vi "Flight Timer.vi"(10 "Aircraft Speed (m/s)":dbl, 11 "System Status":string) -> (2 "Flight Time":string, 3 "Flight Time":dbl)   [LabVIEW 2014]
uses:
  Controls/Flight Timer States.ctl
  Missions/FGVs/Current Mission Distance/Methods/Get Mission Distance.vi
  Missions/FGVs/Virtual Waypoints/Methods/Get Virtual Waypoints.vi
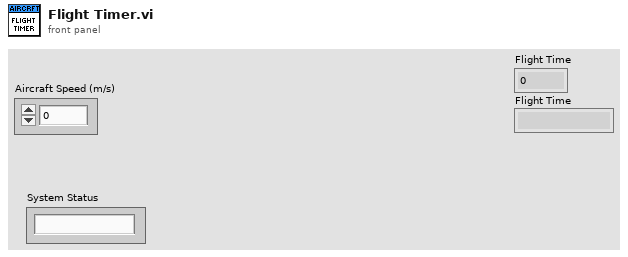
[diagram p1: front panel]
types:
  T1 = typedef "Flight Timer States.ctl" = enum16{"Landed", "Airborne", "Reset Timer"}
  T2 = typedef "Virtual Waypoint.ctl" = cluster{"Waypoint Type":T3, "Lat":sgl, "Lon":sgl, "Altitude (m)":sgl, "Inspection Height (m)":sgl, "Circumnavigate Radius (m)":sgl, "Grid Waypoint?":bool, "Capture Photo":bool, "Speed (m/s)":sgl}
  T3 = typedef "Waypoint Type.ctl" = enum16{"PASS-THROUGH", "INSPECT", "CIRCUMNAVIGATE"}
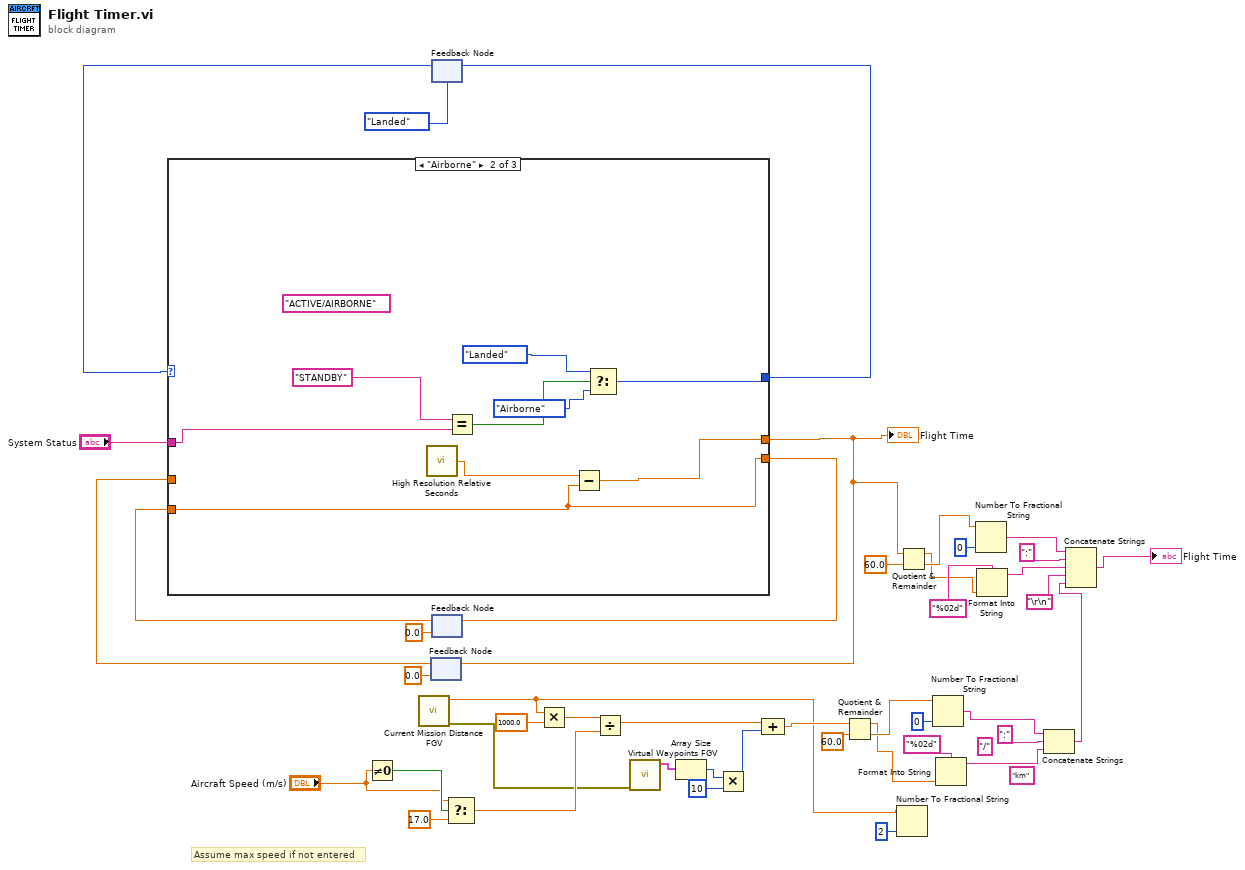
[diagram p0: block diagram]
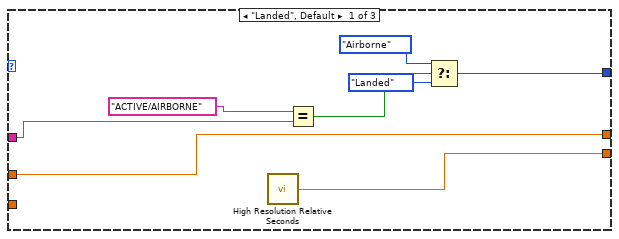
[diagram p2: hidden frame]
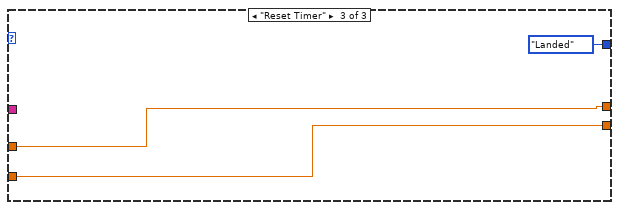
[diagram p3: hidden frame]
diagram:
  (unwired) "km" ("string")
  (unwired) "/" ("string")
  # "Assume max speed if not entered"
  n1 = Not Equal To 0?(x="Aircraft Speed (m/s)") -> (x != 0?=w14:bool)
  n2 = call-poly "Current Mission Distance FGV.vi"() -> ("Error Out"=w1:errorcluster, "Distance Out (km)"=w5:dbl)  [unwired: 10 in]
  n3 = feedback #1(0.0) -> (w38:dbl)
  n4 = feedback #2(Flight_Timer_States."Landed" ("Flight Timer States")) -> (w44:T1)
  n5 = feedback #3(0.0 ("relative seconds")) -> (w41:dbl)
  n6 = case shown="\"Airborne\"" w44 {
    tunnel: "System Status" -> [w51 w60 _]
    tunnel: [w52 w57 w62] -> w42
    tunnel: w41 -> [_ w57 w62]
    tunnel: [w47 w59 Flight_Timer_States."Landed" ("f")] -> w39
    tunnel: [w46 w56 w63] -> w35
    tunnel: w38 -> [w46 _ w63]
    frame "Landed", Default {
      n7 = call <vilib>:"High Resolution Relative Seconds.vi"() -> ("relative seconds"=w52:dbl)
      n8 = Equal?(x="ACTIVE/AIRBORNE", y=w51) -> (x = y?=w49:bool)
      n9 = Select(t=Flight_Timer_States."Airborne", s=w49, f=Flight_Timer_States."Landed") -> (s? t:f=w47:T1)
    }
    frame "Airborne" {
      (unwired) "ACTIVE/AIRBORNE"
      n10 = call <vilib>:"High Resolution Relative Seconds.vi"() -> ("relative seconds"=w58:dbl)
      n11 = Equal?(x="STANDBY", y=w60) -> (x = y?=w61:bool)
      n12 = Subtract(x=w58, y=w57) -> (x-y=w56:dbl)
      n13 = Select(t=Flight_Timer_States."Landed" ("f"), s=w61, f=Flight_Timer_States."Airborne" ("t")) -> (s? t:f=w59:T1)
    }
    frame "Reset Timer" {
    }
  }
  "Flight Time" <- w35
  n14 = feedback-in #1(w35) -> ()
  n15 = feedback-in #2(w39) -> ()
  n16 = feedback-in #3(w42) -> ()
  n17 = Select(t="Aircraft Speed (m/s)", s=w14, f=17.0) -> (s? t:f=w12:dbl)
  n18 = Multiply(x=w5, y=1000.0) -> (x*y=w28:dbl)
  n19 = Divide(x=w28, y=w12) -> (x/y=w7:dbl)
  n20 = call-poly "Virtual Waypoints FGV.vi"("Error In"=w1) -> ("Virtual Waypoints Out"=w10:T2[])  [unwired: 9 in, 1 out]
  n21 = Array Size(array=w10) -> (size(s)=w9:i32)
  n22 = Multiply(x=w9, y=10) -> (x*y=w6:i32)
  n23 = Compound Arithmetic op=ADD(w7, w6) -> (w27:dbl)
  n24 = Quotient & Remainder(x=w27, y=60.0) -> (x-y*floor(x/y)=w17:dbl, floor(x/y)=w24:dbl)
  n25 = Number To Fractional String(number=w5, precision (6)=i16 2) -> ()  [unwired: 2 in, 1 out]
  n26 = Quotient & Remainder(x=w35, y=60.0) -> (x-y*floor(x/y)=w18:dbl, floor(x/y)=w30:dbl)
  n27 = Number To Fractional String(number=w24, precision (6)=i16 0) -> (F-format string=w22:string)  [unwired: 2 in]
  n28 = Format Into String(format string="%02d", w17) -> (resulting string=w16:string)  [unwired: 2 in, 1 out]
  n29 = Number To Fractional String(number=w30, precision (6)=i16 0) -> (F-format string=w33:string)  [unwired: 2 in]
  n30 = Format Into String(format string="%02d", w18) -> (resulting string=w19:string)  [unwired: 2 in, 1 out]
  n31 = Concatenate Strings(w22, ":" ("string"), w16) -> (w2:string)
  n32 = Concatenate Strings(w33, ":" ("string"), w19, "\r\n", w2) -> (→"Flight Time":string)
